vi "TDC_DAQV32_Paralled_muon.vi"(7 "address":string[](array[string])=["192.168.10.20"], 8 "error in (no error)":errorcluster, 9 "stop":bool=TRUE, 10 "save data":bool=TRUE, 11 "SMA mode":bool=TRUE) -> (0 "error out 3":errorcluster, 2 "csv path":path=path "G:/tdc/2017/data/test_20250326_071915.csv", 3 "rate":dbl=0.8977001365215763)   [LabVIEW 2017]
uses:
  gloabal.vi
  <vilib>/Utility/file.llb/Write Delimited Spreadsheet (DBL).vi
  <vilib>/Utility/file.llb/Write Delimited Spreadsheet (I64).vi
panel:
  in  "append csv 2":bool=TRUE
  out "accumulation":u32[][](array[numeric])
  out "pmt trigger rate":u32[](array[numeric])=[42662, 42662, 42662, 42662, 42662, 42662, 42662, 42662, 42662, 42662, 42662, 42662, 42662, 42662, 42662, 42662, 42662, 42662, 42662, 42662, 42662, 42662, 42662, 42662, 42662, 42662, 42662, 42662, 42662, 42662, 42662, 42662, 42662, 42662, 42662, 42662, 42662, 42662, 42662, 42662, 42662, 42662, 42662, 42662, 42662, 42662, 42662, 42662, 42662, 42662, 42662, 42662, 42662, 42662, 42662, 42662, 42662, 42662, 42662, 42662, 42662, 42662, 42662, 42662]
  out "event":u32[](array[numeric])=[26391, 26391, 26391, 26391, 26391, 26391, 26391, 26391, 26391, 26391, 26391, 26391, 26391, 26391, 26391, 26391, 26391, 26391, 26391, 26391, 26391, 26391, 26391, 26391, 26390, 26390, 26390, 26390, 26390, 26390, 26390, 26390, 26390, 26390, 26390, 26390, 26390, 26390, 26390, 26390, 26390, 26390, 26390, 26390, 26390, 26390, 26390, 26390, 26390, 26390, 26390, 26390, 26390, 26390, 26390, 26390, 26390, 26390, 26390, 26390, 26390, 26390, 26390, 26390, 26390, 26390, 26390, 26390, 26390, 26390, 26390, 26390, 26390, 26390, 26390, 26390, 26390, 26390, 26390, 26390, 26390, 26390, 26390, 26390, 26390, 26390, 26390, 26390, 26390, 26390, 26390, 26390, 26390, 26390, 26390, 26390, 26390, 26390, 26390, 26390, 26390, 26390, 26390, 26390, 26390, 26390, 26390, 26390, 26390, 26390, 26390, 26390, 26390, 26390, 26390, 26390, 26390, 26390, 26390, 26390, 26390, 26390, 26390, 26390, 26390, 26390, 26390, 26390]
  in  "calib_file":path=path "G:/tdc/2017/data/test_20250313_032748_codeDensity.csv" caption="文件路径 （空时为对话框）"
  in  "use_calib_file":bool
  out "cal 3":u32[](graph)=[0, 0, 0, 0, 0, 0, 0, 0, 0, 0, 0, 0, 0, 0, 0, 0, 0, 0, 0, 0, 0, 0, 0, 0, 0, 0, 0, 0, 0, 0, 0, 0, 0, 0, 0, 0, 0, 0, 0, 0, 0, 0, 0, 0, 0, 0, 0, 0, 0, 0, 0, 0, 0, 0, 0, 0, 0, 0, 0, 0, 0, 0, 0, 0, 0, 0, 0, 0, 0, 0, 0, 0, 0, 0, 0, 0, 0, 0, 0, 0, 0, 0, 0, 0, 0, 0, 0, 0, 0, 0, 0, 0, 0, 0, 0, 0, 0, 0, 0, 0, 0, 0, 0, 0, 0, 0, 0, 0, 0, 0, 0, 0, 0, 0, 0, 0, 0, 0, 0, 0, 0, 0, 0, 0, 0, 0, 0, 0, 0, 0, 0, 0, 0, 0, 0, 0, 0, 0, 0, 0, 0, 0, 0, 0, 0, 0, 0, 0, 0, 0, 0, 0, 0, 0, 0, 0, 0, 0, 0, 0, 0, 0, 0, 0, 0, 15, 3, 1, 14, 3, 31, 20, 16, 6, 1, 18, 12, 4, 29, 10, 8, 29, 2, 14, 4, 25, 7, 24, 4, 0, 1, 5, 8, 18, 22, 0, 4, 5, 0, 12, 9, 9, 20, 21, 4, 10, 13, 5, 21, 13, 14, 2, 6, 13, 1, 3, 5, 10, 20, 2, 3, 4, 3, 4, 2, 20, 13, 2, 5, 1, 3, 12, 4, 1, 14, 7, 5, 4, 1, 10, 2, 21, 14, 2, 5, 10, 4, 0, 11, 19, 6, 4, 1, 37, 1, 4, 2, 1, 10, 13, 4, 8, 10, 6, 9, 2, 0, 6, 8, 12, 3, 21, 5, 7, 8, 2, 3, 7, 17, 6, 5, 6, 4, 6, 0, 2, 1, 3, 10, 33, 7, 2, 6, 3, 7, 3, 2, 0, 12, 10, 11, 13, 13, 7, 3, 9, 6, 16, 0, 13, 5, 6, 3, 0, 5, 5, 7, 1, 10, 7, 13, 14, 5, 1, 12, 7, 1, 10, 2, 1, 14, 18, 13, 11, 4, 6, 9, 22, 11, 9, 2, 2, 8, 14, 4, 4, 6, 12, 13, 3, 9, 5, 5, 1, 5, 11, 18, 3, 0, 5, 4, 6, 7, 6, 1, 13, 5, 1, 2, 2, 1, 4, 12, 7, 3, 2, 3, 9, 11, 1, 20, 3, 4, 5, 5, 3, 5, 8, 5, 3, 26, 14, 6, 1, 3, 12, 12, 4, 23, 10, 3, 4, 4, 10, 3, 5, 4, 2, 14, 5, 15, 20, 1, 5, 1, 20, 6, 1, 3, 13, 21, 12, 7, 4, 1, 5, 30, 11, 2, 4, 0, 12, 7, 10, 3, 2, 25, 6, 1, 3, 6, 3, 8, 37, 4, 6, 2, 2, 4, 3, 5, 6, 13, 6, 9, 22, 1, 3, 7, 7, 4, 8, 33, 2, 1, 15, 3, 8, 23, 21, 2, 2, 27, 13, 3, 5, 10, 4, 18, 5, 5, 8, 0, 1, 8, 12, 4, 3, 0, 4, 8, 4, 7, 4, 2, 11, 13, 3, 0, 7, 5, 3, 4, 8, 4, 20, 2, 13, 4, 8, 6, 17, 4, 2, 1, 15, 2, 15, 5, 19, 0, 4, 15, 4, 16, 11, 1, 16, 4, 6, 6, 5, 7, 3, 9, 15, 3, 6, 3, 13, 5, 7, 3, 27, 2, 0, 21, 1, 4, 1, 4, 5, 3, 10, 7, 3, 6, 4, 18, 21, 7, 6, 7, 7, 12, 6, 9, 8, 11, 12, 13, 2, 2, 5, 4, 7, 52, 3, 5, 8, 7, 10, 4, 4, 6, 5, 18, 0, 3, 6, 1, 9, 5, 19, 13, 24, 12, 4, 4, 15, 6, 41, 3, 8, 5, 17, 26, 8, 7, 20, 2, 5, 12, 10, 10, 12, 9, 17, 6, 3, 1, 5, 3, 7, 8, 4, 10, 5, 10, 7, 1, 2, 14, 7, 25, 3, 0, 0, 0, 5, 21, 8, 14, 4, 10, 2, 3, 2, 4, 8, 12, 3, 6, 8, 3, 4, 3, 20, 5, 6, 7, 8, 11, 2, 8, 6, 5, 15, 17, 10, 10, 3, 3, 9, 18, 7, 7, 3, 5, 5, 5, 2, 2, 2, 4, 1, 0, 42, 3, 14, 4, 3, 5, 2, 7, 4, 2, 7, 5, 22, 4, 3, 17, 3, 5, 8, 19, 7, 5, 0, 3, 4, 10, 1, 8, 2, 2, 13, 23, 4, 9, 5, 0, 0, 0, 27, 2, 16, 11, 15, 3, 0, 18, 2, 8, 29, 19, 6, 7, 2, 6, 12, 1, 13, 2, 7, 5, 11, 8, 5, 6, 6, 19, 2, 4, 0, 7, 22, 13, 3, 7, 3, 8, 11, 0, 3, 26, 6, 5, 5, 6, 4, 10, 17, 16, 4, 3, 4, 3, 4, 21, 8, 10, 10, 7, 0, 9, 9, 2, 10, 10, 2, 9, 9, 4, 14, 5, 5, 4, 18, 6, 3, 0, 4, 1, 20, 2, 33, 4, 1, 2, 1, 20, 6, 3, 11, 10, 2, 1, 13, 9, 6, 1, 0, 0, 0, 0, 0, 0, 0, 0, 0, 0, 0, 0, 0, 0, 0, 0, 0, 0, 0, 0, 0, 0, 0, 0, 0, 0, 0, 0, 0, 0, 0, 0, 0, 0, 0, 0, 0, 0, 0, 0, 0, 0, 0, 0, 0, 0, 0, 0, 0, 0, 0, 0, 0, 0, 0, 0, 0, 0, 0, 0, 0, 0, 0, 0, 0, 0, 0, 0, 0, 0, 0, 0, 0, 0, 0, 0, 0, 0, 0, 0, 0, 0, 0, 0, 0, 0, 0, 0, 0, 0, 0, 0, 0, 0, 0, 0, 0, 0, 0, 0, 0, 0, 0, 0, 0, 0, 0, 0, 0, 0, 0, 0, 0, 0, 0, 0, 0, 0, 0, 0, 0, 0, 0, 0, 0, 0, 0, 0, 0, 0, 0, 0, 0, 0, 0, 0, 0, 0, 0, 0, 0, 0, 0, 0, 0, 0, 0, 0, 0, 0, 0, 0, 0, 0, 0, 0, 0, 0, 0, 0, 0, 0, 0, 0, 0, 0, 0, 0, 0, 0, 0, 0, 0, 0, 0, 0, 0, 0, 0, 0, 0, 0, 0, 0, 0, 0, 0, 0, 0, 0, 0, 0, 0, 0, 0, 0, 0, 0, 0, 0, 0, 0, 0, 0, 0, 0, 0, 0, 0, 0, 0, 0, 0, 0, 0, 0, 0, 0, 0, 0, 0, 0, 0, 0, 0, 0, 0, 0, 0, 0, 0, 0, 0, 0, 0, 0, 0, 0, 0, 0, 0, 0, 0, 0, 0, 0, 0, 0, 0, 0, 0, 0, 0, 0, 0, 0, 0, 0, 0, 0, 0, 0, 0, 0, 0, 0, 0, 0, 0, 0, 0, 0, 0, 0, 0, 0, 0, 0, 0, 0, 0, 0, 0, 0, 0, 0, 0, 0, 0, 0, 0, 0, 0, 0, 0, 0, 0, 0, 0, 0, 0, 0, 0, 0, 0, 0, 0, 0, 0, 0, 0, 0, 0, 0, 0, 0, 0, 0, 0, 0, 0, 0, 0, 0, 0, 0, 0, 0, 0, 0, 0, 0, 0, 0, 0, 0, 0, 0, 0, 0, 0, 0, 0, 0, 0, 0, 0, 0, 0, 0, 0, 0, 0, 0, 0, 0, 0, 0, 0, 0, 0, 0, 0, 0, 0, 0, 0, 0, 0, 0, 0, 0, 0, 0, 0, 0, 0, 0, 0, 0, 0, 0, 0, 0, 0, 0, 0, 0, 0, 0, 0, 0, 0, 0, 0, 0, 0, 0, 0, 0, 0, 0, 0, 0, 0, 0, 0, 0, 0, 0, 0, 0, 0, 0, 0, 0, 0, 0, 0, 0, 0, 0, 0, 0, 0, 0, 0, 0, 0, 0, 0, 0, 0, 0, 0, 0, 0, 0, 0, 0, 0, 0, 0, 0, 0, 0, 0, 0, 0, 0, 0, 0, 0, 0, 0, 0, 0, 0, 0, 0, 0, 0, 0, 0, 0, 0, 0, 0, 0, 0, 0, 0, 0, 0, 0, 0, 0, 0, 0, 0, 0, 0, 0, 0, 0, 0, 0, 0, 0, 0, 0, 0, 0, 0, 0, 0, 0, 0, 0, 0, 0, 0, 0, 0, 0, 0, 0, 0, 0, 0, 0, 0, 0, 0, 0, 0, 0, 0, 0, 0, 0, 0, 0, 0, 0, 0, 0, 0, 0, 0, 0, 0, 0, 0, 0, 0, 0, 0, 0, 0, 0, 0, 0, 0, 0, 0, 0, 0, 0, 0, 0, 0, 0, 0, 0, 0, 0, 0, 0, 0, 0, 0, 0, 0, 0, 0, 0, 0, 0, 0, 0, 0, 0, 0, 0, 0, 0, 0, 0, 0, 0, 0, 0, 0, 0, 0, 0, 0, 0, 0, 0, 0, 0, 0, 0, 0, 0, 0, 0, 0, 0, 0, 0, 0, 0, 0, 0, 0, 0, 0, 0, 0, 0, 0, 0, 0, 0, 0, 0, 0, 0, 0, 0, 0, 0, 0, 0, 0, 0, 0, 0, 0, 0, 0, 0, 0, 0, 0, 0, 0, 0, 0, 0, 0, 0, 0, 0, 0, 0, 0, 0, 0, 0, 0, 0, 0, 0, 0, 0, 0, 0, 0, 0, 0, 0, 0, 0, 0, 0, 0, 0, 0, 0, 0, 0, 0, 0, 0, 0, 0, 0, 0, 0, 0, 0, 0, 0, 0, 0, 0, 0, 0, 0, 0, 0, 0, 0, 0, 0, 0, 0, 0, 0, 0, 0, 0, 0, 0, 0, 0, 0, 0, 0, 0, 0, 0, 0, 0, 0, 0, 0, 0, 0, 0, 0, 0, 0, 0, 0, 0, 0, 0, 0, 0, 0, 0, 0, 0, 0, 0, 0, 0, 0, 0, 0, 0, 0, 0, 0, 0, 0, 0, 0, 0, 0, 0, 0, 0, 0, 0, 0, 0, 0, 0, 0, 0, 0, 0, 0, 0, 0, 0, 0, 0, 0, 0, 0, 0, 0, 0, 0, 0, 0, 0, 0, 0, 0, 0, 0, 0, 0, 0, 0, 0, 0, 0, 0, 0, 0, 0, 0, 0, 0, 0, 0, 0, 0, 0, 0, 0, 0, 0, 0, 0, 0, 0, 0, 0, 0, 0, 0, 0, 0, 0, 0, 0, 0, 0, 0, 0, 0, 0, 0, 0, 0, 0, 0, 0, 0, 0, 0, 0, 0, 0, 0, 0, 0, 0, 0, 0, 0, 0, 0, 0, 0, 0, 0, 0, 0, 0, 0, 0, 0, 0, 0, 0, 0, 0, 0, 0, 0, 0, 0, 0, 0, 0, 0, 0, 0, 0, 0, 0, 0, 0, 0, 0, 0, 0, 0, 0, 0, 0, 0, 0, 0, 0, 0, 0, 0, 0, 0, 0, 0, 0, 0, 0, 0, 0, 0, 0, 0, 0, 0, 0, 0, 0, 0, 0, 0, 0, 0, 0, 0, 0, 0, 0, 0, 0, 0, 0, 0, 0, 0, 0, 0, 0, 0, 0, 0, 0, 0, 0, 0, 0, 0, 0, 0, 0, 0, 0, 0, 0, 0, 0, 0, 0, 0, 0, 0, 0, 0, 0, 0, 0, 0, 0, 0, 0, 0, 0, 0, 0, 0, 0, 0, 0, 0, 0, 0, 0, 0, 0, 0, 0, 0, 0, 0, 0, 0, 0, 0, 0, 0, 0, 0, 0, 0, 0, 0, 0, 0, 0, 0, 0, 0, 0, 0, 0, 0, 0, 0, 0, 0, 0, 0, 0, 0, 0, 0, 0, 0, 0, 0, 0, 0, 0, 0, 0, 0, 0, 0, 0, 0, 0, 0, 0, 0, 0, 0, 0, 0, 0, 0, 0, 0, 0, 0, 0, 0, 0, 0, 0, 0, 0, 0, 0, 0, 0, 0, 0, 0, 0, 0, 0, 0, 0, 0, 0, 0, 0, 0, 0, 0, 0, 0, 0, 0, 0, 0, 0, 0, 0, 0, 0, 0, 0, 0, 0, 0, 0, 0, 0, 0, 0, 0, 0, 0, 0, 0, 0, 0, 0, 0, 0, 0, 0, 0, 0, 0, 0, 0, 0, 0, 0, 0, 0, 0, 0, 0, 0, 0, 0, 0, 0, 0, 0, 0, 0, 0, 0, 0, 0, 0, 0, 0, 0, 0, 0, 0, 0, 0, 0, 0, 0, 0, 0, 0, 0, 0, 0, 0, 0, 0, 0, 0, 0, 0, 0, 0, 0, 0, 0, 0, 0, 0, 0, 0, 0, 0, 0, 0, 0, 0, 0, 0, 0, 0, 0, 0, 0, 0, 0, 0, 0, 0, 0, 0, 0, 0, 0, 0, 0, 0, 0, 0, 0, 0, 0, 0, 0, 0, 0, 0, 0, 0, 0, 0, 0, 0, 0, 0, 0, 0, 0, 0, 0, 0, 0, 0, 0, 0, 0, 0, 0, 0]
  out "second stamp":u64
  in  "coarse counter width":u16(ring) items=["29", "48"]
  out "name (unnamed)":string
  out "error out 5":errorcluster
  in  "timeout":dbl=30000.0
  out "DAC":dbl=8094.0
  out "Out":u8=3 format="%.0x"
  out "coarse":u64=454674664 format="%x"
  in  "gps":bool
  out "Year":string="2025"
  in  "factor":i32=128
  in  "displayCR":bool=TRUE
  in  "Counter Setting":dbl=100000.0 format="%#_13g"
  in  "replace dat":bool
  in  "append csv":bool=TRUE
  out "element":string
  out "fine":u64=621 format="%x"
  in  "UDP Config":bool=TRUE
  in  "data  path":path=path "G:/tdc/2017/data"
  out "cal 2":u64[](graph)
  in  "Thresholds (mV)":dbl[](array[numeric])=[580.0, 580.0, 580.0, 580.0, 600.0, 600.0, 600.0, 600.0, 580.0, 580.0, 600.0, 600.0, 600.0, 600.0, 600.0, 600.0, 580.0, 580.0, 600.0, 600.0, 600.0, 600.0, 600.0, 600.0, 580.0, 580.0, 600.0, 600.0, 600.0, 600.0, 600.0, 600.0, 600.0, 600.0, 600.0, 600.0, 600.0, 600.0, 600.0, 600.0, 600.0, 600.0, 600.0, 600.0, 600.0, 600.0, 600.0, 600.0, 600.0, 600.0, 600.0, 600.0, 600.0, 600.0, 600.0, 600.0, 600.0, 600.0, 600.0, 600.0, 600.0, 600.0, 600.0, 600.0]
  out "error out 2":errorcluster
  in  "display":bool=TRUE
  in  "Thresholds":dbl=-0.03
  in  "one key for threshold":bool=TRUE
  in  "RST":bool
  in  "通道数量":i32=128
  out "Cal Table":u32[](array[numeric])=[100002, 100002, 100002, 100002, 100002, 100002, 100002, 100002, 100002, 100002, 100002, 100002, 100002, 100002, 100002, 100002, 100002, 100002, 100002, 100002, 100002, 100002, 100002, 100002, 100002, 100002, 100002, 100002, 100002, 100002, 100002, 100002, 100002, 100002, 100002, 100002, 100002, 100002, 100002, 100002, 100002, 100002, 100002, 100002, 100002, 100002, 100002, 100002, 100002, 100002, 100002, 100002, 100002, 100002, 100002, 100002, 100002, 100002, 100002, 100002, 100002, 100002, 100002, 100002, 100002, 100002, 100002, 100002, 100002, 100002, 100002, 100002, 100002, 100002, 100002, 100002, 100002, 100002, 100002, 100002, 100002, 100002, 100002, 100002, 100002, 100002, 100002, 100002, 100002, 100002, 100002, 100002, 100002, 100002, 100002, 100002, 100002, 100002, 100002, 100002, 100002, 100002, 100002, 100002, 100002, 100002, 100002, 100002, 100002, 100002, 100002, 100002, 100002, 100002, 100002, 100002, 100002, 100002, 100002, 100002, 100002, 100002, 100002, 100002, 100002, 100002, 100002, 100002]
  in  "channel for cal":i32
  out "channel number":u64
  out "Calibration Counter":i32=100000
  out "Event index":i32=97959
  out "cal":i64[](graph)=[0, 0, 0, 0, 0, 0, 0, 0, 0, 0, 0, 0, 0, 0, 0, 0, 0, 0, 0, 0, 0, 0, 0, 0, 0, 0, 0, 0, 0, 0, 0, 0, 0, 0, 0, 0, 0, 0, 0, 0, 0, 0, 0, 0, 0, 0, 0, 0, 0, 0, 0, 0, 0, 0, 0, 0, 0, 0, 0, 0, 0, 0, 0, 0, 0, 0, 0, 0, 0, 0, 0, 0, 0, 0, 0, 0, 0, 0, 0, 0, 0, 0, 0, 0, 0, 0, 0, 0, 0, 0, 0, 0, 0, 0, 0, 0, 0, 0, 0, 0, 0, 0, 0, 0, 0, 0, 0, 0, 0, 0, 0, 0, 0, 0, 0, 0, 0, 0, 0, 0, 0, 0, 0, 0, 0, 0, 0, 0, 0, 0, 0, 0, 0, 0, 0, 0, 0, 0, 0, 470, 444, 62, 95, 368, 213, 276, 85, 576, 217, 42, 61, 213, 135, 123, 54, 784, 126, 136, 66, 62, 275, 126, 450, 146, 386, 84, 83, 84, 62, 253, 57, 502, 202, 53, 85, 337, 200, 58, 83, 413, 78, 317, 61, 148, 133, 102, 48, 479, 56, 216, 194, 40, 112, 63, 351, 135, 190, 64, 93, 227, 93, 232, 114, 257, 110, 101, 159, 65, 42, 76, 54, 50, 44, 34, 359, 299, 101, 217, 71, 56, 60, 35, 455, 55, 67, 165, 158, 73, 196, 324, 124, 309, 54, 58, 141, 218, 413, 311, 78, 256, 130, 114, 294, 134, 50, 55, 28, 324, 26, 45, 329, 65, 45, 61, 116, 74, 323, 82, 79, 76, 85, 71, 72, 82, 187, 243, 204, 247, 62, 155, 92, 292, 69, 301, 30, 91, 225, 164, 64, 174, 87, 39, 48, 55, 627, 68, 232, 183, 142, 127, 63, 54, 315, 53, 77, 55, 116, 317, 193, 216, 219, 230, 235, 57, 55, 234, 42, 47, 57, 143, 358, 59, 153, 234, 79, 52, 154, 36, 378, 66, 258, 119, 74, 244, 119, 148, 52, 254, 251, 157, 243, 71, 102, 77, 477, 87, 292, 296, 458, 55, 177, 38, 31, 35, 56, 381, 340, 362, 127, 55, 39, 79, 277, 44, 40, 62, 68, 250, 24, 117, 88, 162, 67, 344, 104, 160, 92, 123, 54, 92, 68, 278, 168, 79, 408, 53, 38, 58, 56, 61, 51, 226, 81, 206, 224, 500, 85, 60, 69, 185, 271, 118, 166, 51, 65, 152, 192, 52, 91, 90, 286, 93, 314, 82, 82, 106, 261, 208, 80, 229, 101, 81, 224, 153, 256, 98, 36, 59, 67, 613, 43, 43, 40, 267, 68, 56, 271, 170, 98, 131, 79, 159, 86, 165, 217, 404, 83, 71, 135, 94, 174, 172, 48, 56, 441, 218, 102, 71, 139, 121, 137, 130, 148, 401, 140, 150, 182, 72, 207, 72, 62, 128, 217, 156, 471, 148, 53, 39, 329, 106, 142, 164, 131, 231, 54, 182, 112, 141, 281, 153, 313, 69, 72, 41, 181, 218, 56, 141, 81, 198, 63, 58, 241, 203, 104, 45, 40, 47, 205, 84, 42, 44, 387, 216, 158, 43, 59, 146, 97, 73, 100, 342, 95, 83, 88, 277, 184, 104, 53, 65, 275, 156, 245, 83, 62, 118, 206, 283, 48, 91, 102, 173, 63, 398, 66, 132, 65, 188, 274, 51, 53, 168, 132, 106, 221, 49, 50, 103, 174, 71, 211, 557, 53, 102, 53, 204, 86, 150, 145, 68, 211, 44, 81, 420, 104, 142, 288, 175, 62, 71, 473, 67, 134, 127, 170, 74, 65, 146, 161, 79, 106, 142, 273, 138, 369, 67, 79, 180, 264, 83, 430, 55, 98, 97, 181, 45, 247, 290, 174, 330, 59, 190, 39, 34, 33, 58, 203, 128, 109, 108, 82, 293, 87, 62, 98, 103, 58, 52, 46, 712, 43, 50, 133, 458, 172, 395, 40, 43, 159, 147, 158, 109, 667, 52, 38, 107, 336, 421, 194, 61, 296, 123, 176, 103, 87, 166, 71, 165, 673, 92, 58, 171, 158, 64, 62, 120, 117, 207, 128, 149, 55, 63, 80, 137, 395, 136, 100, 110, 227, 70, 132, 142, 66, 113, 419, 55, 35, 62, 201, 78, 444, 318, 150, 54, 241, 72, 45, 54, 112, 201, 339, 87, 74, 279, 84, 136, 156, 98, 295, 59, 372, 94, 109, 76, 101, 122, 109, 209, 266, 83, 153, 259, 425, 131, 78, 229, 112, 66, 144, 47, 42, 125, 91, 418, 268, 143, 61, 36, 57, 219, 95, 46, 200, 120, 424, 116, 180, 252, 147, 184, 183, 76, 123, 180, 296, 531, 86, 54, 63, 173, 311, 698, 101, 76, 70, 106, 88, 275, 465, 105, 160, 48, 44, 88, 334, 497, 123, 42, 60, 34, 296, 72, 68, 73, 141, 259, 79, 46, 57, 60, 92, 72, 9, 21, 0, 0, 0, 0, 0, 0, 0, 0, 0, 0, 0, 0, 0, 0, 0, 0, 0, 0, 0, 0, 0, 0, 0, 0, 0, 0, 0, 0, 0, 0, 0, 0, 0, 0, 0, 0, 0, 0, 0, 0, 0, 0, 0, 0, 0, 0, 0, 0, 0, 0, 0, 0, 0, 0, 0, 0, 0, 0, 0, 0, 0, 0, 0, 0, 0, 0, 0, 0, 0, 0, 0, 0, 0, 0, 0, 0, 0, 0, 0, 0, 0, 0, 0, 0, 0, 0, 0, 0, 0, 0, 0, 0, 0, 0, 0, 0, 0, 0, 0, 0, 0, 0, 0, 0, 0, 0, 0, 0, 0, 0, 0, 0, 0, 0, 0, 0, 0, 0, 0, 0, 0, 0, 0, 0, 0, 0, 0, 0, 0, 0, 0, 0, 0, 0, 0, 0, 0, 0, 0, 0, 0, 0, 0, 0, 0, 0, 0, 0, 0, 0, 0, 0, 0, 0, 0, 0, 0, 0, 0, 0, 0, 0, 0, 0, 0, 0, 0, 0, 0, 0, 0, 0, 0, 0, 0, 0, 0, 0, 0, 0, 0, 0, 0, 0, 0, 0, 0, 0, 0, 0, 0, 0, 0, 0, 0, 0, 0, 0, 0, 0, 0, 0, 0, 0, 0, 0, 0, 0, 0, 0, 0, 0, 0, 0, 0, 0, 0, 0, 0, 0, 0, 0, 0, 0, 0, 0, 0, 0, 0, 0, 0, 0, 0, 0, 0, 0, 0, 0, 0, 0, 0, 0, 0, 0, 0, 0, 0, 0, 0, 0, 0, 0, 0, 0, 0, 0, 0, 0, 0, 0, 0, 0, 0, 0, 0, 0, 0, 0, 0, 0, 0, 0, 0, 0, 0, 0, 0, 0, 0, 0, 0, 0, 0, 0, 0, 0, 0, 0, 0, 0, 0, 0, 0, 0, 0, 0, 0, 0, 0, 0, 0, 0, 0, 0, 0, 0, 0, 0, 0, 0, 0, 0, 0, 0, 0, 0, 0, 0, 0, 0, 0, 0, 0, 0, 0, 0, 0, 0, 0, 0, 0, 0, 0, 0, 0, 0, 0, 0, 0, 0, 0, 0, 0, 0, 0, 0, 0, 0, 0, 0, 0, 0, 0, 0, 0, 0, 0, 0, 0, 0, 0, 0, 0, 0, 0, 0, 0, 0, 0, 0, 0, 0, 0, 0, 0, 0, 0, 0, 0, 0, 0, 0, 0, 0, 0, 0, 0, 0, 0, 0, 0, 0, 0, 0, 0, 0, 0, 0, 0, 0, 0, 0, 0, 0, 0, 0, 0, 0, 0, 0, 0, 0, 0, 0, 0, 0, 0, 0, 0, 0, 0, 0, 0, 0, 0, 0, 0, 0, 0, 0, 0, 0, 0, 0, 0, 0, 0, 0, 0, 0, 0, 0, 0, 0, 0, 0, 0, 0, 0, 0, 0, 0, 0, 0, 0, 0, 0, 0, 0, 0, 0, 0, 0, 0, 0, 0, 0, 0, 0, 0, 0, 0, 0, 0, 0, 0, 0, 0, 0, 0, 0, 0, 0, 0, 0, 0, 0, 0, 0, 0, 0, 0, 0, 0, 0, 0, 0, 0, 0, 0, 0, 0, 0, 0, 0, 0, 0, 0, 0, 0, 0, 0, 0, 0, 0, 0, 0, 0, 0, 0, 0, 0, 0, 0, 0, 0, 0, 0, 0, 0, 0, 0, 0, 0, 0, 0, 0, 0, 0, 0, 0, 0, 0, 0, 0, 0, 0, 0, 0, 0, 0, 0, 0, 0, 0, 0, 0, 0, 0, 0, 0, 0, 0, 0, 0, 0, 0, 0, 0, 0, 0, 0, 0, 0, 0, 0, 0, 0, 0, 0, 0, 0, 0, 0, 0, 0, 0, 0, 0, 0, 0, 0, 0, 0, 0, 0, 0, 0, 0, 0, 0, 0, 0, 0, 0, 0, 0, 0, 0, 0, 0, 0, 0, 0, 0, 0, 0, 0, 0, 0, 0, 0, 0, 0, 0, 0, 0, 0, 0, 0, 0, 0, 0, 0, 0, 0, 0, 0, 0, 0, 0, 0, 0, 0, 0, 0, 0, 0, 0, 0, 0, 0, 0, 0, 0, 0, 0, 0, 0, 0, 0, 0, 0, 0, 0, 0, 0, 0, 0, 0, 0, 0, 0, 0, 0, 0, 0, 0, 0, 0, 0, 0, 0, 0, 0, 0, 0, 0, 0, 0, 0, 0, 0, 0, 0, 0, 0, 0, 0, 0, 0, 0, 0, 0, 0, 0, 0, 0, 0, 0, 0, 0, 0, 0, 0, 0, 0, 0, 0, 0, 0, 0, 0, 0, 0, 0, 0, 0, 0, 0, 0, 0, 0, 0, 0, 0, 0, 0, 0, 0, 0, 0, 0, 0, 0, 0, 0, 0, 0, 0, 0, 0, 0, 0, 0, 0, 0, 0, 0, 0, 0, 0, 0, 0, 0, 0, 0, 0, 0, 0, 0, 0, 0, 0, 0, 0, 0, 0, 0, 0, 0, 0, 0, 0, 0, 0, 0, 0, 0, 0, 0, 0, 0, 0, 0, 0, 0, 0, 0, 0, 0, 0, 0, 0, 0, 0, 0, 0, 0, 0, 0, 0, 0, 0, 0, 0, 0, 0, 0, 0, 0, 0, 0, 0, 0, 0, 0, 0, 0, 0, 0, 0, 0, 0, 0, 0, 0, 0, 0, 0, 0, 0, 0, 0, 0, 0, 0, 0, 0, 0, 0, 0, 0, 0, 0, 0, 0, 0, 0, 0, 0, 0, 0, 0, 0, 0, 0, 0, 0, 0, 0, 0, 0, 0, 0, 0, 0, 0, 0, 0, 0, 0, 0, 0, 0, 0, 0, 0, 0, 0, 0, 0, 0, 0, 0, 0, 0, 0, 0, 0, 0, 0, 0, 0, 0, 0, 0, 0, 0, 0, 0, 0, 0, 0, 0, 0, 0, 0, 0, 0, 0, 0, 0, 0, 0, 0, 0, 0, 0, 0, 0, 0, 0, 0, 0, 0, 0, 0, 0, 0, 0, 0, 0, 0, 0, 0, 0, 0, 0, 0, 0, 0, 0, 0, 0, 0, 0, 0, 0, 0, 0, 0, 0, 0, 0, 0, 0, 0, 0, 0, 0, 0, 0, 0, 0, 0, 0, 0, 0, 0, 0, 0, 0, 0, 0, 0, 0, 0, 0, 0, 0, 0, 0, 0, 0, 0, 0, 0, 0, 0, 0, 0, 0, 0, 0, 0, 0, 0, 0, 0, 0, 0, 0, 0, 0, 0, 0, 0, 0, 0, 0, 0, 0, 0, 0, 0, 0, 0, 0, 0, 0, 0, 0, 0, 0, 0, 0, 0, 0, 0, 0, 0, 0, 0, 0, 0, 0, 0, 0, 0, 0, 0, 0, 0, 0, 0, 0, 0, 0, 0, 0, 0, 0, 0, 0, 0, 0, 0, 0, 0, 0, 0, 0, 0, 0, 0, 0, 0, 0, 0, 0, 0, 0, 0, 0, 0, 0, 0, 0, 0, 0, 0, 0, 0, 0, 0, 0, 0, 0, 0, 0, 0, 0, 0, 0, 0, 0, 0, 0, 0, 0, 0, 0, 0, 0, 0, 0, 0, 0, 0, 0, 0, 0, 0, 0, 0, 0, 0, 0, 0, 0, 0, 0, 0, 0, 0, 0, 0, 0, 0, 0, 0, 0, 0, 0, 0, 0, 0, 0, 0, 0, 0, 0, 0, 0, 0, 0, 0, 0, 0, 0, 0, 0, 0, 0, 0, 0, 0, 0, 0, 0, 0, 0, 0, 0, 0, 0, 0, 0, 0, 0, 0, 0, 0, 0, 0, 0, 0, 0, 0, 0, 0, 0, 0, 0, 0, 0, 0, 0, 0, 0, 0, 0, 0, 0, 0, 0, 0, 0, 0, 0, 0, 0, 0, 0, 0, 0, 0, 0, 0, 0, 0, 0, 0, 0, 0, 0, 0, 0, 0, 0, 0, 0, 0, 0, 0, 0, 0, 0, 0, 0, 0, 0, 0, 0, 0, 0, 0, 0, 0, 0, 0, 0, 0, 0, 0, 0, 0, 0, 0, 0, 0, 0, 0]
  out "error out":errorcluster
  out "appended path":path=path "G:/tdc/2017/data/test_20250326_071915.dat"
  in  "filename":string="test"
  in  "Events":i32=110000 min=1
  in  "timeout (ms)":i32=10000
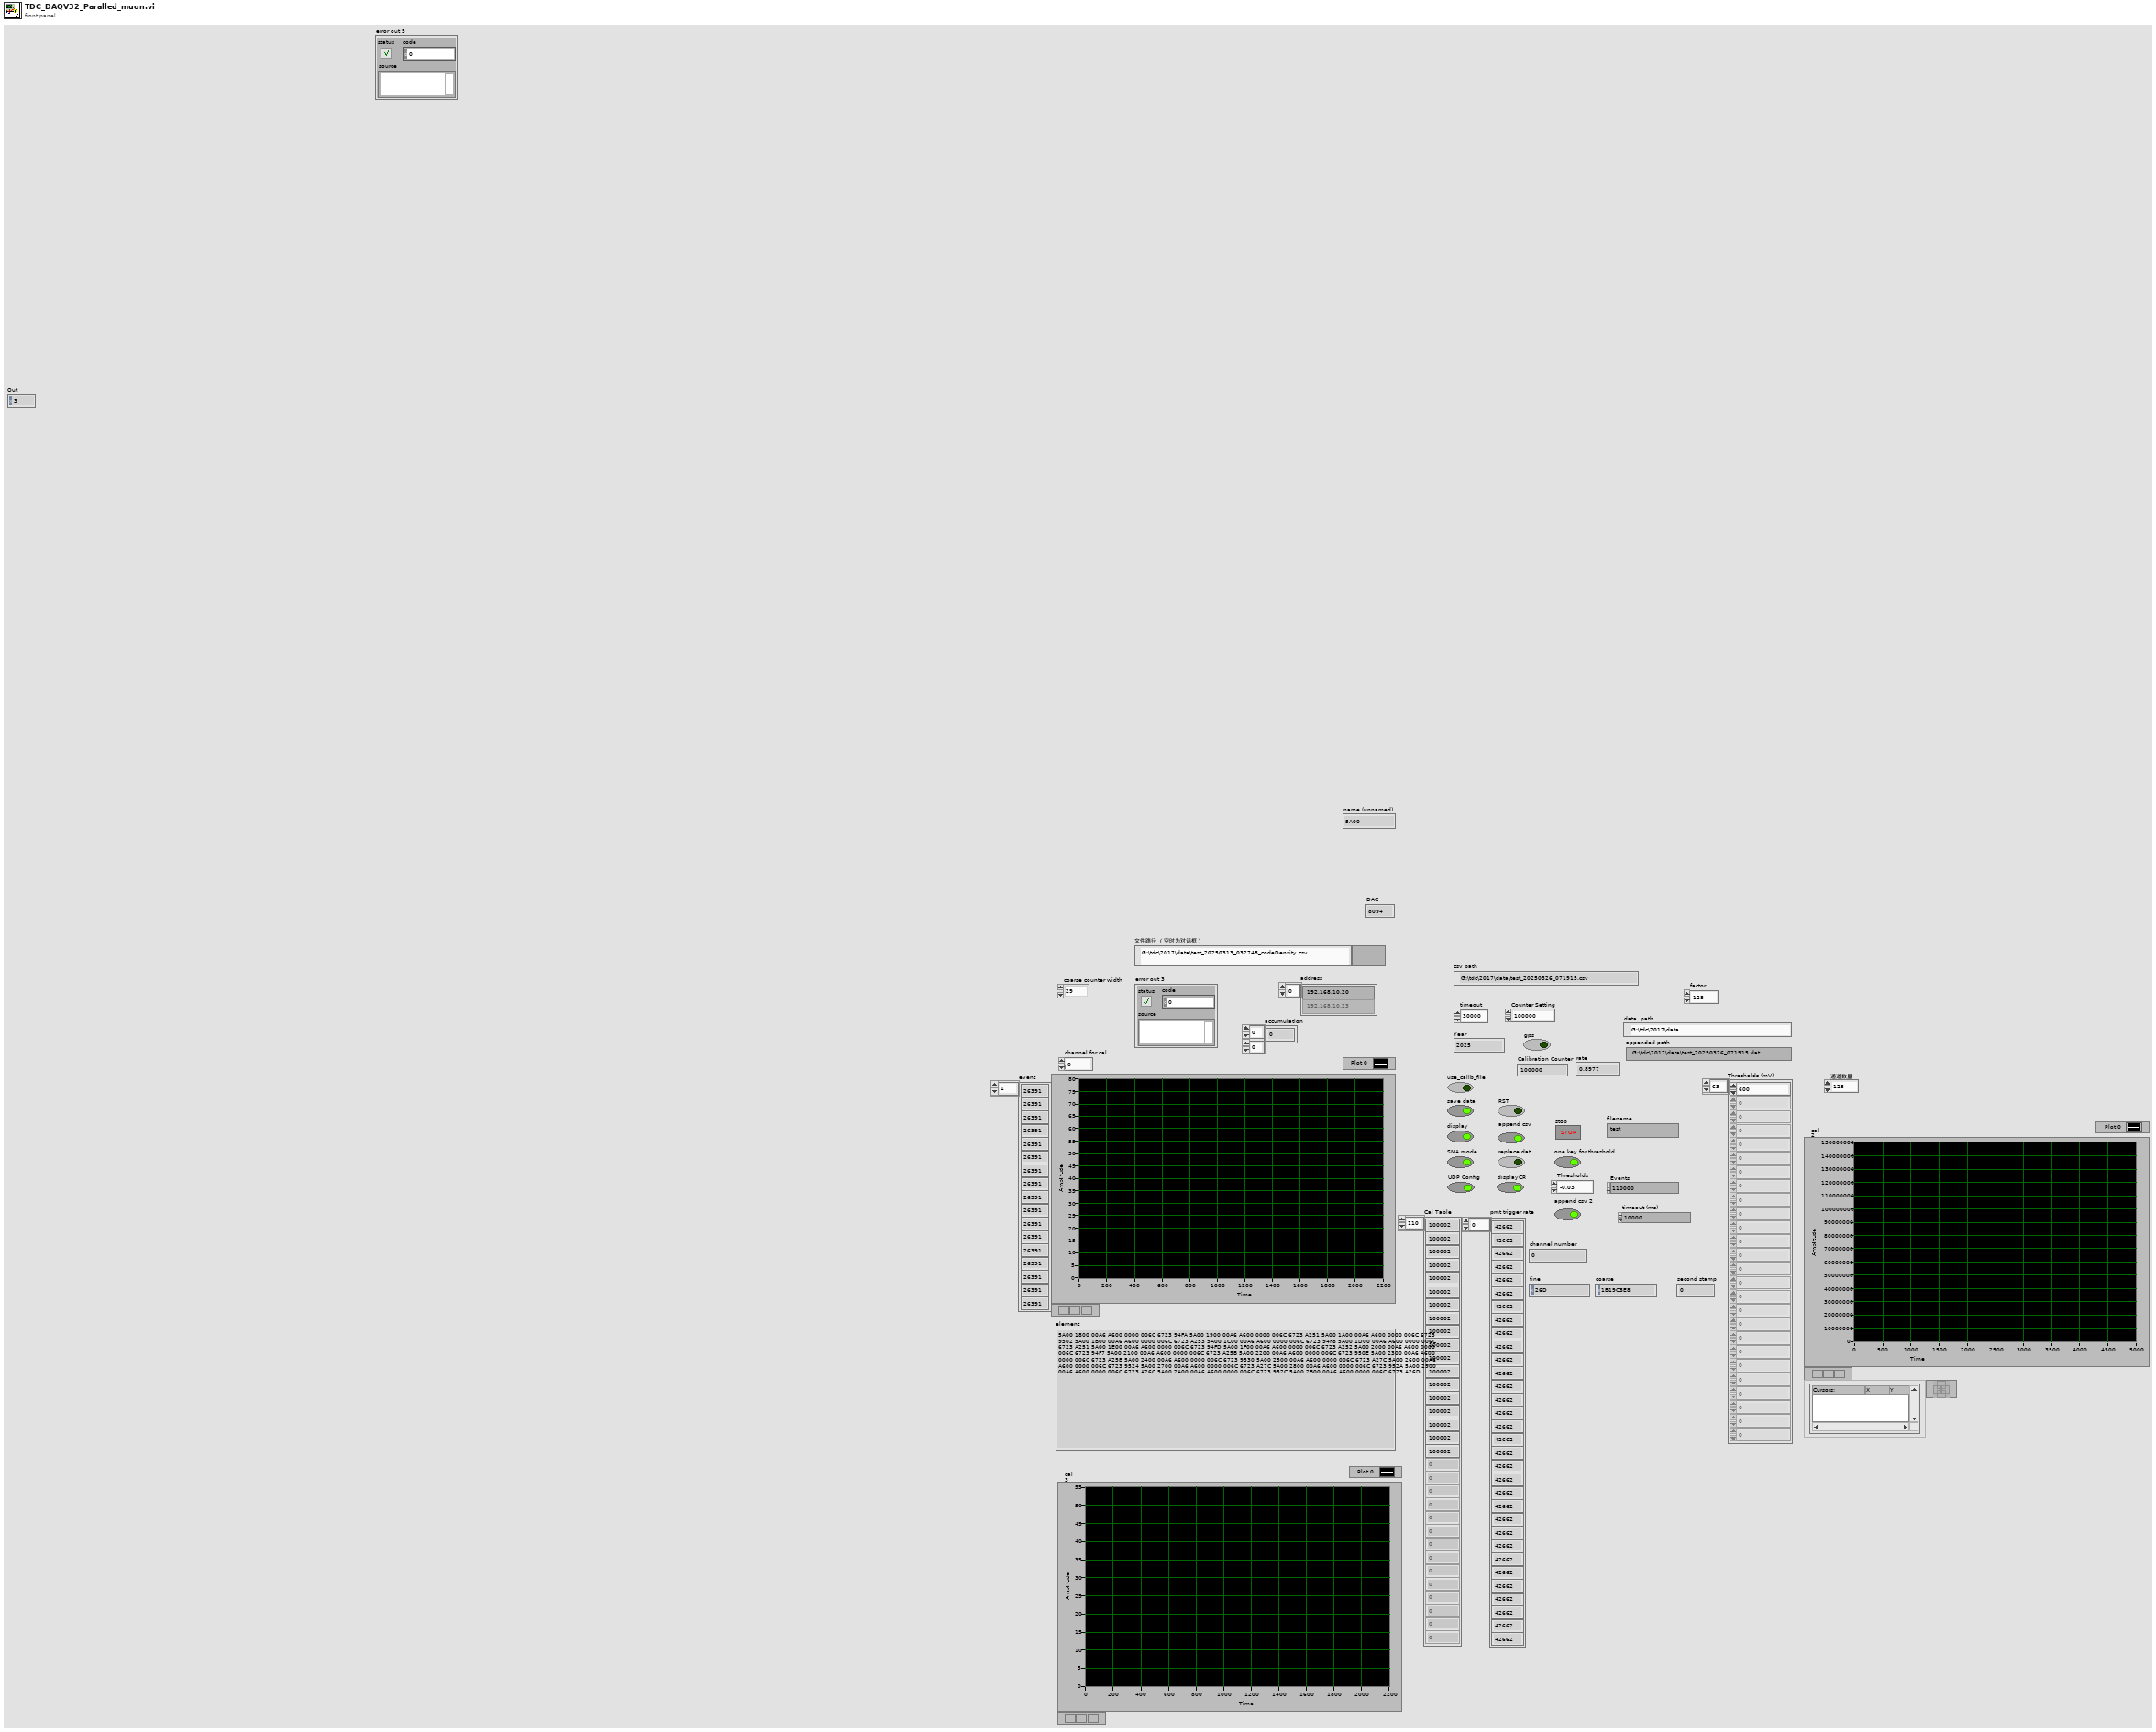
[diagram p1: front panel]
types:
  T1 = enum16{"open", "replace", "create", "open or create", "replace or create", "replace or create with confirmation"}
  T2 = enum16{"big-endian, network order", "native, host order", "little-endian"}
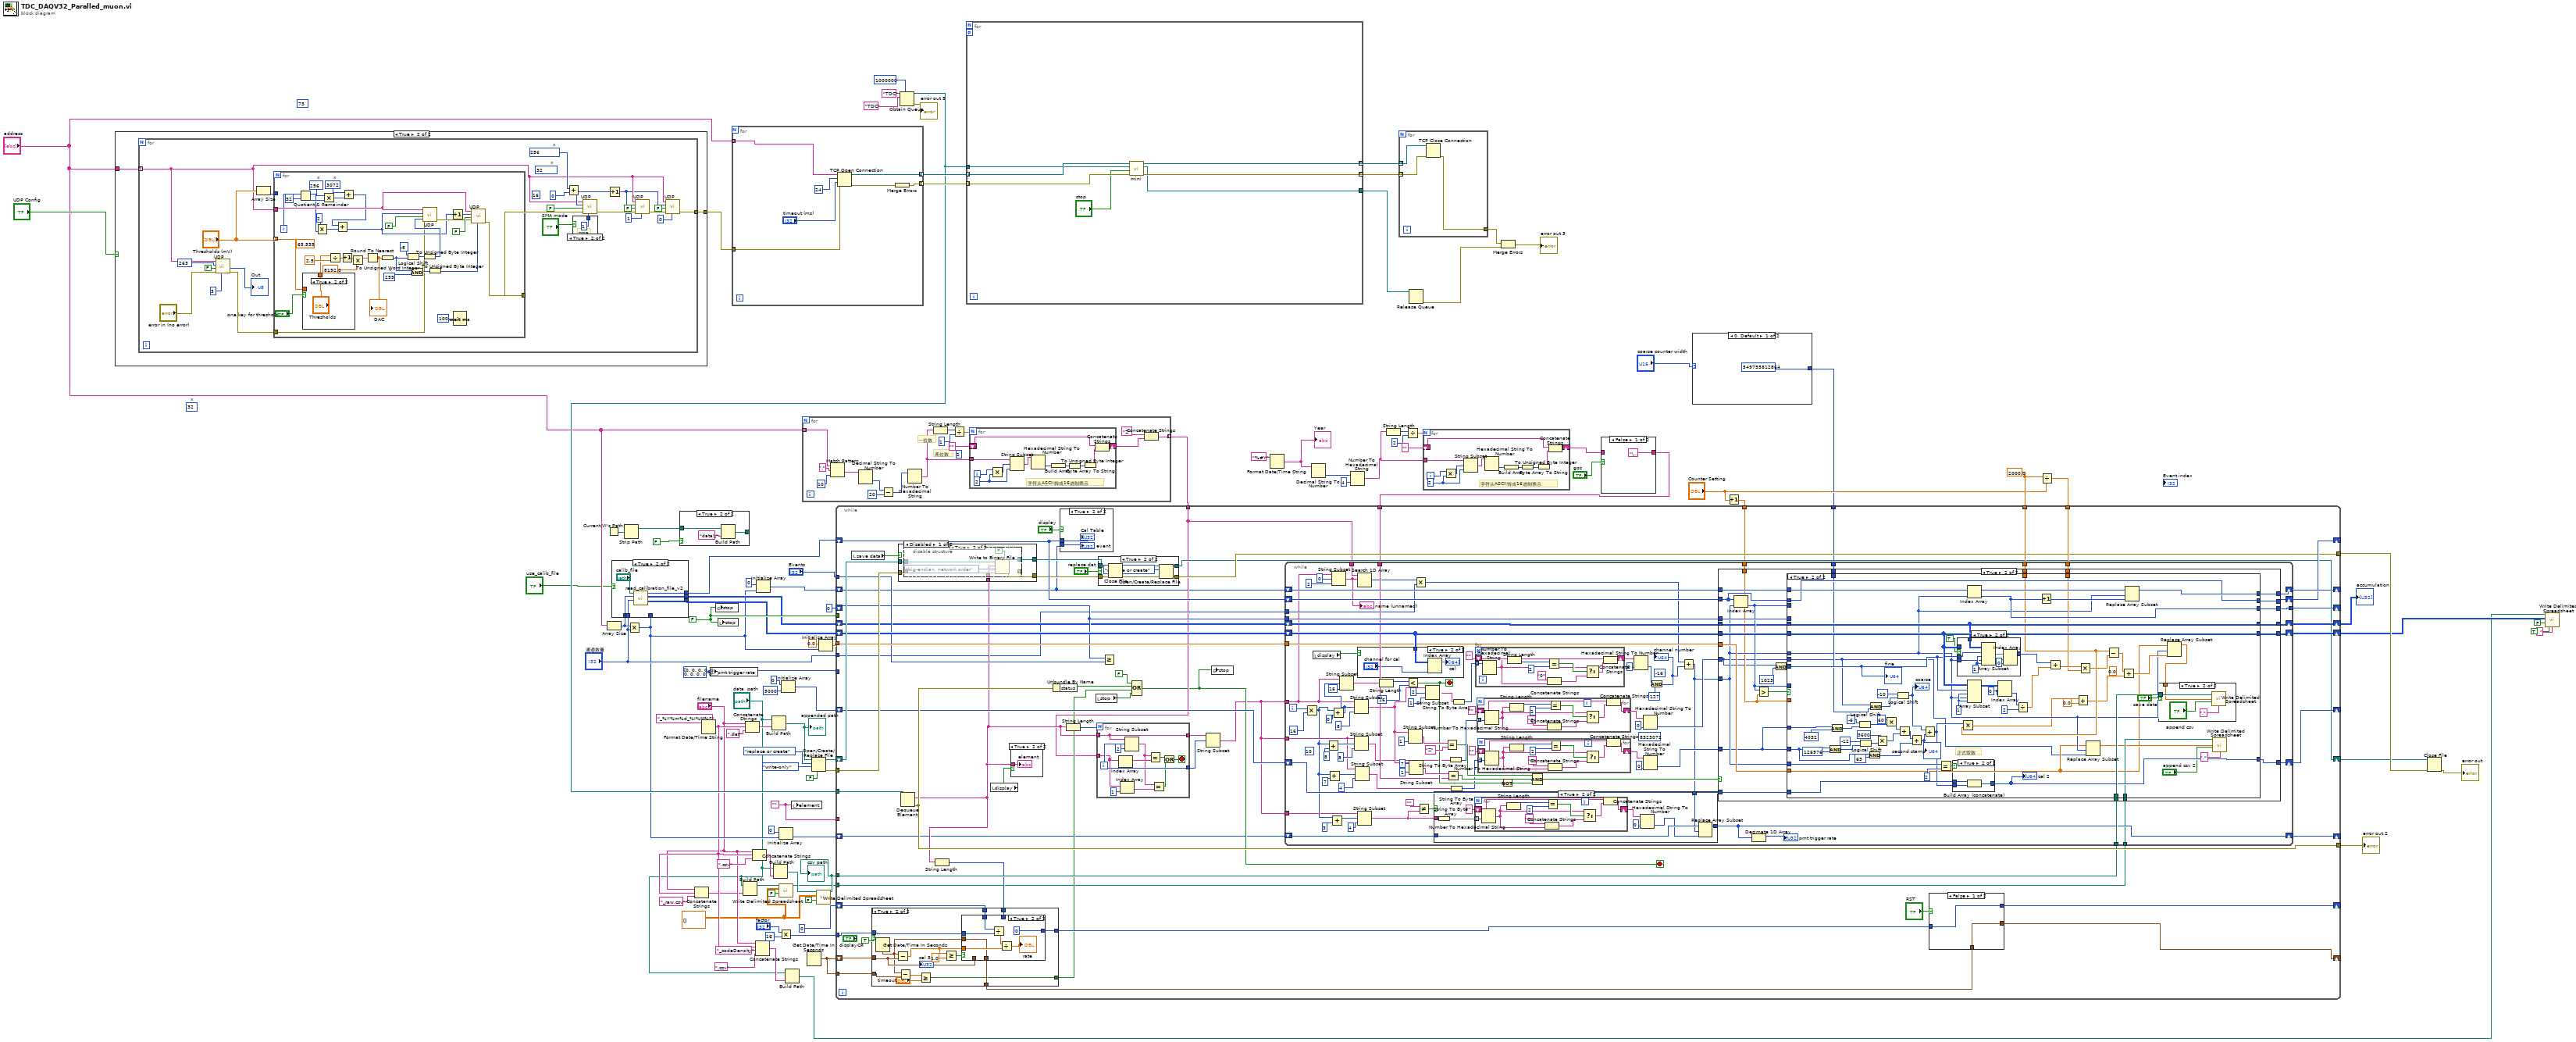
[diagram p0: block diagram]
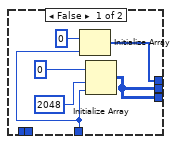
[diagram p2: hidden frame]
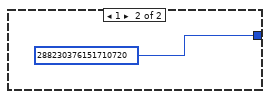
[diagram p3: hidden frame]
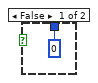
[diagram p6: hidden frame]
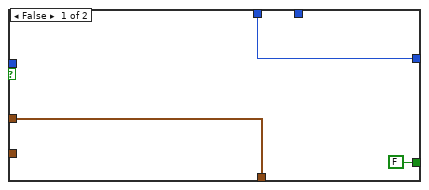
[diagram p13: hidden frame]
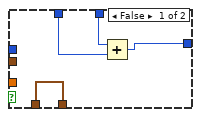
[diagram p14: hidden frame]
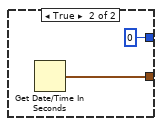
[diagram p16: hidden frame]
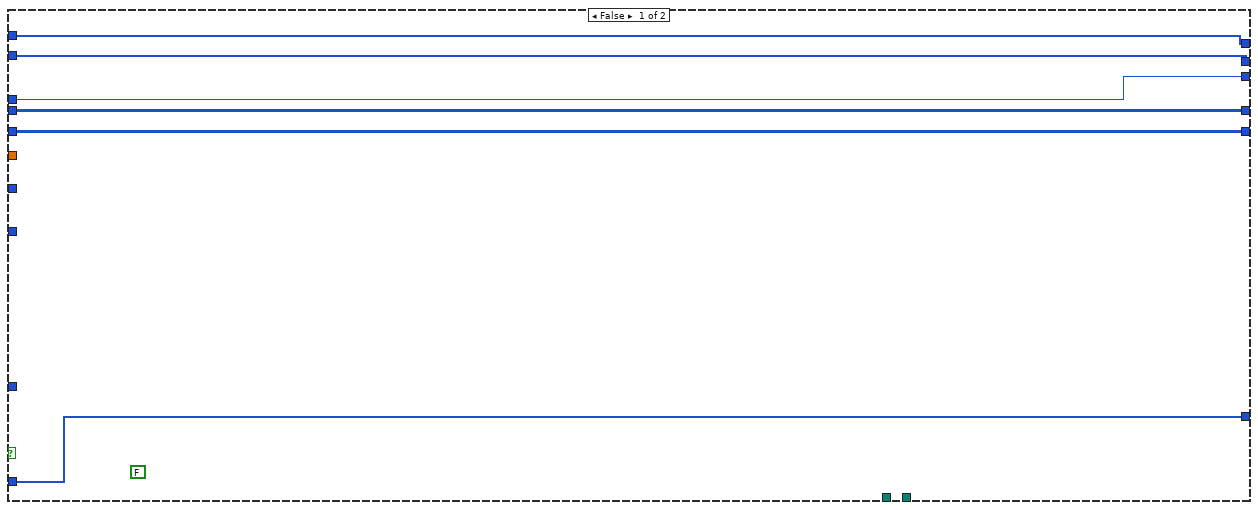
[diagram p19: hidden frame]
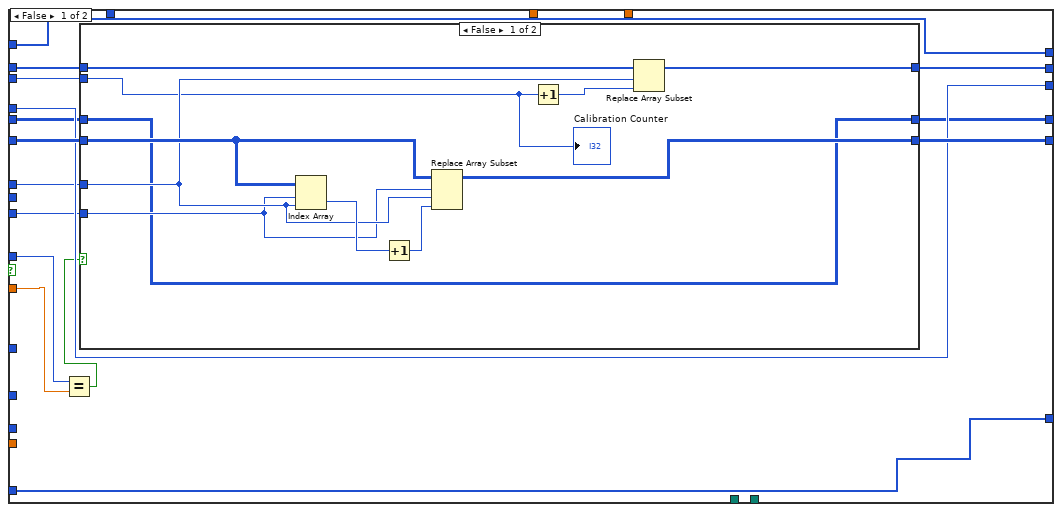
[diagram p20: hidden frame]
diagram:
  w11 = ""
  w12 = u32[] [0, 0, 0, 0, 0, 0, 0, 0, 0, 0, 0, 0, 0, 0, 0, 0, 0, 0, 0, 0, 0, 0, 0, 0, 0, 0, 0, 0, 0, 0, 0, 0, 0, 0, 0, 0, 0, 0, 0, 0, 0, 0, 0, 0, 0, 0, 0, 0, 0, 0, 0, 0, 0, 0, 0, 0, 0, 0, 0, 0, 0, 0, 0, 0] ("pmt trigger rate")
  (unwired) u32 73 ("Address")
  w63 = 2000.0 ("x")
  (unwired) u16 32  # x
  w25 = FALSE ("stop")
  w4 = dbl[][] [] ("2D data")
  n1 = case shown="True" "UDP Config" {
    tunnel: "address" -> [_ w101]
    tunnel: [_ w102] -> w30
    frame False {
    }
    frame True {
      n2 = for {
        tunnel: [w107] -> w102
        tunnel: w101 -> [w105] mode=indexing
        (unwired) u16 32  # x
        (unwired) u32 16 ("Address")
        w119 = u16 256  # x
        n3 = call "UDP.vi"("In"=u8 3, "error in (no error)"="error in (no error)", "Read (TRUE)"=FALSE, "Address"=u32 263, "IP address"=w105) -> ("error out"=w113:errorcluster, "Out"=→"Out":u8)  [unwired: 3 in, 1 out]
        n4 = Array Size(array="Thresholds (mV)") -> (size(s)=w122:i32)
        n5 = for {
          tunnel: w105 -> [w158]
          tunnel: "Thresholds (mV)" -> [w145] mode=indexing
          tunnel: [w148] -> w125
          tunnel: w122 -> [_]
          tunnel: w113 -> [w132]
          i -> [w140]
          (unwired) 65.535 ("y")
          w141 = u16 3072  # x
          w142 = u16 256  # x
          w154 = u16 255  # x
          n6 = Quotient & Remainder(x=w140, y=32) -> (x-y*floor(x/y)=w134:i32, floor(x/y)=w143:i32)
          n7 = case shown="True" "one key for threshold" {
            tunnel: [w164 "Thresholds"] -> w146
            tunnel: w145 -> [w164 _]
            frame False {
            }
            frame True {
            }
          }
          n8 = Multiply(x=2, y=w134) -> (x*y=w135:i32)
          n9 = Multiply(x=w142, y=w143) -> (x*y=w137:i32)
          n10 = Divide(x=w146, y=2.5) -> (x/y=w161:dbl)
          n11 = Increment(x=w161) -> (x+1=w131:dbl)
          n12 = Add(x=w141, y=w137) -> (x+y=w136:i32)
          n13 = Add(x=w136, y=w135) -> (x+y=w139:i32)
          n14 = Multiply(x=w131, y=8192.0) -> (x*y=w130:dbl)
          n15 = Round To Nearest(number=w130) -> (nearest integer value=w159:dbl)
          "DAC" <- w159
          n16 = To Unsigned Word Integer(number=w159) -> (unsigned 16bit integer=w150:u16)
          n17 = Logical Shift(y=i16 -8, x=w150) -> (x << y=w156:u16)
          n18 = And(x=w150, y=w154) -> (x .and. y?=w153:u16)
          n19 = To Unsigned Byte Integer(number=w156) -> (unsigned 8bit integer=w155:u8)
          n20 = call "UDP.vi"("In"=w155, "error in (no error)"=w132, "Read (TRUE)"=FALSE, "Address"=w139, "IP address"=w158) -> ("error out"=w149:errorcluster)  [unwired: 3 in, 2 out]
          n21 = To Unsigned Byte Integer(number=w153) -> (unsigned 8bit integer=w152:u8)
          n22 = Increment(x=w139) -> (x+1=w138:i32)
          n23 = Wait (ms)(milliseconds to wait=u32 100) -> ()  [unwired: 1 out]
          n24 = call "UDP.vi"("In"=w152, "error in (no error)"=w149, "Read (TRUE)"=FALSE, "Address"=w138, "IP address"=w158) -> ("error out"=w148:errorcluster)  [unwired: 3 in, 2 out]
        }
        n25 = Add(x=w119, y=u32 0 ("Address")) -> (x+y=w111:u32)
        n26 = case shown="True" "SMA mode" {
          tunnel: [u8 0 ("In") u8 1 ("In")] -> w124
          frame False {
          }
          frame True {
            # "sma"
          }
        }
        n27 = call "UDP.vi"("In"=w124, "error in (no error)"=w125, "Read (TRUE)"=FALSE, "Address"=w111, "IP address"=w105) -> ("error out"=w112:errorcluster)  [unwired: 3 in, 2 out]
        n28 = Increment(x=w111) -> (x+1=w104:u32)
        n29 = call "UDP.vi"("In"=u8 1, "error in (no error)"=w112, "Read (TRUE)"=FALSE, "Address"=w104, "IP address"=w105) -> ("error out"=w108:errorcluster)  [unwired: 3 in, 2 out]
        n30 = call "UDP.vi"("In"=u8 0, "error in (no error)"=w108, "Read (TRUE)"=FALSE, "Address"=w104, "IP address"=w105) -> ("error out"=w107:errorcluster)  [unwired: 3 in, 2 out]
      }
    }
  }
  n31 = Current VI's Path() -> (path=w95:path)
  n32 = Array Size(array="address") -> (size(s)=w17:i32)
  n33 = Strip Path(path=w95) -> (stripped path=w94:path)  [unwired: 1 out]
  n34 = Multiply(x=w17, y="通道数量") -> (x*y=w14:i32)
  n35 = case shown="True" "use_calib_file" {
    tunnel: w14 -> [w169 _]
    tunnel: [w166 w177] -> w20
    tunnel: [w166 w176] -> w19
    tunnel: [w167 w175] -> w18
    tunnel: w17 -> [_ w174]
    tunnel: "通道数量" -> [_ w173]
    frame False {
      n36 = Initialize Array(u32 0 ("element"), w169) -> (w167:u32[])
      n37 = Initialize Array(u32 0 ("element"), 2048 ("dimension size"), w169) -> (w166:u32[][])
    }
    frame True {
      n38 = call "read_calibration_file_v2.vi"("通道数量"=w173, "板子数量"=w174, "file path (dialog if empty)"="calib_file") -> ("code_density"=w177:i64[][], "accumulation"=w176:u32[][], "Cal Table"=w175:u32[])  [unwired: 5 in, 1 out]
    }
  }
  n39 = case shown="True" FALSE {
    tunnel: w94 -> [w178 w180]
    tunnel: [w178 w179] -> _
    frame False {
    }
    frame True {
      n40 = Build Path(base path=w180, name or relative path="data\\") -> (appended path=w179:path)
    }
  }
  n41 = Format Date/Time String(time format string (%c)="_%Y%m%d_%I%M%S") -> (date/time string=w8:string)  [unwired: 2 in]
  n42 = Concatenate Strings("filename", w8, "_raw.csv") -> (w6:string)
  n43 = local write "pmt trigger rate"(w12) -> ()
  n44 = global write "gloabal.vi" "stop"(w25) -> ()
  n45 = local write "stop"(w25) -> ()
  n46 = for {
    tunnel: "address" -> [w187] mode=indexing
    tunnel: [w186] -> w40 mode=indexing
    tunnel: [w184] -> w39 mode=indexing
    tunnel: w30 -> [w183]
    n47 = TCP Open Connection(address=w187, remote port or service name=u16 24 ("port"), timeout ms (60000)="timeout (ms)", error in (no error)=w183) -> (connection ID=w186:refnum<k5>, error out=w185:errorcluster)  [unwired: 1 in]
    n48 = Merge Errors(w185) -> (w184:errorcluster)
  }
  n49 = Build Path(base path="data  path", name or relative path=w6) -> (appended path=w1:path)
  n50 = Concatenate Strings("filename", w8, ".dat") -> (w93:string)
  n51 = Concatenate Strings("filename", w8, ".csv") -> (w83:string)
  n52 = Concatenate Strings("filename", w8, "_codeDensity" ("string"), ".csv") -> (w76:string)
  n53 = Initialize Array(u32 0 ("element"), w14) -> (w82:u32[])
  n54 = Build Path(base path="data  path", name or relative path=w93) -> (appended path=w92:path)
  "appended path" <- w92
  n55 = Build Path(base path="data  path", name or relative path=w83) -> (appended path=w81:path)
  n56 = Initialize Array(u32 0 ("element"), w14) -> (w13:u32[])
  n57 = call-poly <vilib>:"Write Delimited Spreadsheet.vi"("file path (dialog if empty)"=w1, "2D data"=w4, "append to file? (new file:F)"=FALSE) -> ("new file path (Not A Path if cancelled)"=w2:path)  [unwired: 11 in, 1 out]
  n58 = Multiply(x="factor", y=16) -> (x*y=w56:i32)
  n59 = Initialize Array(u32 0 ("element"), 5000 ("dimension size")) -> (w67:u32[])
  n60 = Build Path(base path="data  path", name or relative path=w76) -> (appended path=w73:path)
  n61 = local write "element"(w11) -> ()
  n62 = for {
    tunnel: [w190] -> w42 mode=indexing
    tunnel: "address" -> [w189] mode=indexing
    (unwired) 2 ("y")
    # "一位数"
    # "两位数"
    n63 = Match Pattern(string=w189, regular expression="." ("search string"), offset (0)=10) -> (after substring=w196:string)  [unwired: 3 out]
    n64 = Decimal String To Number(string=w196) -> (number=w193:i32)  [unwired: 2 in, 1 out]
    n65 = Subtract(x=w193, y=20) -> (x-y=w192:i32)
    n66 = Number To Hexadecimal String(2:w192) -> (0:w195:string)  [unwired: 1 in]
    n67 = String Length(string=w195) -> (length=w201:i32)
    n68 = Divide(x=w201, y=1) -> (x/y=w202:dbl)
    n69 = for {
      N: w202 -> [_]
      shift-right: [w214] -> w191
      shift-left: "" ("format string") -> [w213]
      tunnel: w195 -> [w204]
      i -> [w212]
      w206 = 2 ("y")
      # "字符从ASCII转成16进制表示"
      n70 = Multiply(x=w212, y=w206) -> (x*y=w205:i32)
      n71 = String Subset(string=w204, offset (0)=w205, length (rest)=w206) -> (substring=w207:string)
      n72 = Hexadecimal String To Number(string=w207) -> (number=w211:u32)  [unwired: 2 in, 1 out]
      n73 = Build Array(w211) -> (w210:u32[])
      n74 = To Unsigned Byte Integer(number=w210) -> (unsigned 8bit integer=w209:u8[])
      n75 = Byte Array To String(unsigned byte array=w209) -> (string=w208:string)
      n76 = Concatenate Strings(w213, w208) -> (w214:string)
    }
    n77 = Concatenate Strings("Z", w191) -> (w190:string)
  }
  n78 = Get Date/Time In Seconds() -> (seconds since 1Jan1904=w41:timestamp)
  n79 = Open/Create/Replace File(file path (use dialog)=w92, operation (0:open)=T1."replace or create", access (0:read/write)=enum16{"read/write", "read-only", "write-only"}."write-only", disable buffering (F)=FALSE) -> (refnum out=w97:refnum<file>, error out=w96:errorcluster)  [unwired: 2 in, 1 out]
  n80 = call-poly <vilib>:"Write Delimited Spreadsheet.vi"("file path (dialog if empty)"=w81, "2D data"=w4, "append to file? (new file:F)"=FALSE) -> ("new file path (Not A Path if cancelled)"=w24:path)  [unwired: 11 in, 1 out]
  "csv path" <- w24
  n81 = Initialize Array(0.0, w14) -> (w69:dbl[])
  n82 = Obtain Queue(max queue size (-1, unlimited)=1000000, name (unnamed)="TDC", element data type="TDC" ("name (unnamed)")) -> (queue out=w31:refnum<queue>, error out=→"error out 5":errorcluster)  [unwired: 2 in, 1 out]
  n83 = for {
    tunnel: w40 -> [w221] mode=indexing
    tunnel: w39 -> [w220] mode=indexing
    tunnel: [w219] -> w38 mode=indexing
    tunnel: [w218] -> w37 mode=indexing
    workers-P: _ -> [_]
    tunnel: w31 -> [w217]
    tunnel: [w216] -> w32
    n84 = call "mini.vi"("error in (no error)"=w220, "stop"="stop", "queue out 2"=w217, "connection ID 2"=w221) -> ("error out 3"=w218:errorcluster, "queue out"=w216:refnum<queue>, "connection ID"=w219:refnum<k5>)  [unwired: 5 in]
  }
  n85 = Format Date/Time String(time format string (%c)="%#Y") -> (date/time string=w53:string)  [unwired: 2 in]
  "Year" <- w53
  n86 = Decimal String To Number(string=w53) -> (number=w52:i32)  [unwired: 2 in, 1 out]
  n87 = Number To Hexadecimal String(1:i16 4 ("width (-)"), 2:w52) -> (0:w46:string)
  n88 = String Length(string=w46) -> (length=w48:i32)
  n89 = for {
    tunnel: w38 -> [w224] mode=indexing
    tunnel: w37 -> [w223] mode=indexing
    tunnel: [w222] -> w29
    n90 = TCP Close Connection(connection ID=w224, error in (no error)=w223) -> (error out=w222:errorcluster)  [unwired: 1 in, 1 out]
  }
  n91 = Divide(x=w48, y=2) -> (x/y=w49:dbl)
  n92 = Release Queue(queue=w32) -> (error out=w28:errorcluster)  [unwired: 2 in, 2 out]
  n93 = for {
    N: w49 -> [_]
    shift-right: [w235] -> w45
    shift-left: "" ("format string") -> [w234]
    tunnel: w46 -> [w225]
    i -> [w233]
    w227 = 2 ("y")
    # "字符从ASCII转成16进制表示"
    n94 = Multiply(x=w233, y=w227) -> (x*y=w226:i32)
    n95 = String Subset(string=w225, offset (0)=w226, length (rest)=w227) -> (substring=w228:string)
    n96 = Hexadecimal String To Number(string=w228) -> (number=w232:u32)  [unwired: 2 in, 1 out]
    n97 = Build Array(w232) -> (w231:u32[])
    n98 = To Unsigned Byte Integer(number=w231) -> (unsigned 8bit integer=w230:u8[])
    n99 = Byte Array To String(unsigned byte array=w230) -> (string=w229:string)
    n100 = Concatenate Strings(w234, w229) -> (w235:string)
  }
  n101 = Merge Errors(w29, w28) -> (→"error out 3":errorcluster)
  n102 = case shown="False" "gps" {
    tunnel: w45 -> [_ w237]
    tunnel: ["\u0000" ("format string") w237] -> w44
    frame False {
    }
    frame True {
    }
  }
  n103 = case shown="0, Default" "coarse counter width" {
    tunnel: [u64 549755812864 ("port") u64 288230376151710720 ("port")] -> w22
    frame 0, Default {
    }
    frame 1 {
    }
  }
  n104 = Increment(x="Counter Setting") -> (x+1=w59:dbl)
  n105 = Divide(x=w63, y="Counter Setting") -> (x/y=w62:dbl)
  n106 = while {
    tunnel: w96 -> [w297]
    tunnel: [w278] -> w70
    tunnel: [w267] -> w89
    shift-right: [w294] -> w74
    shift-left: w20 -> [w295]
    tunnel: "Events" -> [w292]
    shift-right: [w291] -> _
    shift-left: w82 -> [w244]
    shift-right: [w290] -> _
    shift-left: u32 0 ("element") -> [w289]
    shift-right: [w288] -> _
    shift-left: w18 -> [w280]
    shift-right: [w282] -> w10
    shift-left: w19 -> [w287]
    tunnel: w24 -> [w274]
    shift-right: [w286] -> _
    shift-left: 0 -> [w261]
    shift-right: [w284] -> _
    shift-left: w41 -> [w283]
    tunnel: w25 -> [_]
    tunnel: w31 -> [w279]
    shift-right: [w275] -> _
    shift-left: w67 -> [w276]
    tunnel: w42 -> [w248]
    tunnel: w63 -> [w272]
    tunnel: w62 -> [w271]
    shift-right: [w266] -> w61
    shift-left: w97 -> [w296]
    tunnel: w59 -> [w265]
    tunnel: w56 -> [w258]
    tunnel: w44 -> [w256]
    tunnel: w41 -> [w255]
    tunnel: "通道数量" -> [w249]
    tunnel: w22 -> [w245]
    shift-right: [w241] -> _
    shift-left: w13 -> [w242]
    tunnel: w12 -> [_]
    tunnel: w11 -> [_]
    tunnel: w2 -> [w240]
    tunnel: w69 -> [w293]
    stop <- w247 stop-if-true
    n107 = local read "save data"() -> (w260:bool)
    n108 = Dequeue Element(queue=w279) -> (element=w251:string, error out=w278:errorcluster)  [unwired: 2 in, 2 out]
    n109 = case shown="True" w260 {
      tunnel: w297 -> [w310 w316]
      tunnel: w296 -> [w311 w315]
      tunnel: w251 -> [_ w314]
      tunnel: [w311 w313] -> w270
      tunnel: [w310 w312] -> w268
      frame False {
      }
      frame True {
        n110 = disable-structure shown="Disabled" {
          disable-tunnel: w316 -> [w323 _]
          disable-tunnel: w315 -> [w322 _]
          disable-tunnel: w314 -> [w319 _]
          disable-tunnel: [w318 _] -> w313
          disable-tunnel: [w317 _] -> w312
          frame Disabled {
            n111 = Write to Binary File(file (use dialog)=w322, data=w319, error in=w323, 5:FALSE ("prepend array or string size? (T)"), 9:T2."big-endian, network order" ("byte order (0:big-endian, network order)")) -> (refnum out=w318:refnum<file>, error out=w317:errorcluster)  [unwired: 1 in, 1 out]
          }
          frame Enabled {
          }
        }
      }
    }
    n112 = String Length(string=w251) -> (length=w262:i32)
    n113 = case shown="True" TRUE {
      tunnel: w283 -> [w335 w345]
      tunnel: [w335 w346] -> w264
      tunnel: w261 -> [w334 w344]
      tunnel: w262 -> [_ w343]
      tunnel: [w334 w342] -> w263
      tunnel: w258 -> [_ w341]
      tunnel: w255 -> [_ w339]
      tunnel: [FALSE w336] -> w254
      frame False {
      }
      frame True {
        n114 = Get Date/Time In Seconds() -> (seconds since 1Jan1904=w340:timestamp)
        n115 = Subtract(x=w340, y=w345) -> (x-y=w348:dbl)
        n116 = Subtract(x=w340, y=w339) -> (x-y=w338:dbl)
        n117 = Greater Or Equal?(x=w338, y="timeout") -> (x >= y?=w336:bool)
        n118 = Greater Or Equal?(x=w348, y=1.0) -> (x >= y?=w349:bool)
        n119 = case shown="True" w349 {
          tunnel: w348 -> [_ w360]
          tunnel: w340 -> [_ w358]
          tunnel: [w353 w358] -> w346
          tunnel: w345 -> [w353 _]
          tunnel: w344 -> [w352 w355]
          tunnel: w343 -> [w351 _]
          tunnel: [w350 0] -> w342
          tunnel: w341 -> [_ w354]
          frame False {
            n120 = Add(x=w351, y=w352) -> (x+y=w350:i32)
          }
          frame True {
            n121 = Divide(x=w355, y=w354) -> (x/y=w357:dbl)
            n122 = Divide(x=w357, y=w360) -> (x/y=→"rate":dbl)
          }
        }
      }
    }
    n123 = local read "display"() -> (w259:bool)
    n124 = case shown="True" w259 {
      tunnel: w251 -> [_ w309]
      frame False {
      }
      frame True {
        "element" <- w309
      }
    }
    n125 = Unbundle By Name(w278) -> ("status"=w277:bool)
    n126 = case shown="True" "display" {
      tunnel: w280 -> [_ w362]
      tunnel: w244 -> [_ w361]
      frame False {
      }
      frame True {
        "Cal Table" <- w362
        "event" <- w361
      }
    }
    n127 = String Length(string=w251) -> (length=w253:i32)
    n128 = local read "stop"() -> (w246:bool)
    n129 = for {
      N: w253 -> [_]
      tunnel: w251 -> [w306]
      tunnel: [w306] -> w252
      tunnel: [w305] -> w250
      tunnel: w248 -> [w303]
      i -> [w305]
      stop <- w299 stop-if-true
      n130 = Index Array(array=w303) -> (element=w304:string)  [unwired: 1 in]
      n131 = Index Array(array=w303, index=1) -> (element=w301:string)
      n132 = String Subset(string=w306, offset (0)=w305, length (rest)=2 ("length (rest)")) -> (substring=w300:string)
      n133 = Equal?(x=w300, y=w304) -> (x = y?=w307:bool)
      n134 = Equal?(x=w300, y=w301) -> (x = y?=w298:bool)
      n135 = Or(x=w307, y=w298) -> (x .or. y?=w299:bool)
    }
    n136 = case shown="True" "replace dat" {
      tunnel: w270 -> [w325 w331]
      tunnel: [w325 w330] -> w266
      tunnel: w268 -> [w324 w327]
      tunnel: [w324 w326] -> w267
      frame False {
      }
      frame True {
        n137 = Close File(refnum=w331, error in=w327) -> (path=w332:path, error out=w328:errorcluster)
        n138 = Open/Create/Replace File(file path (use dialog)=w332, error in=w328, operation (0:open)=T1."replace or create") -> (refnum out=w330:refnum<file>, error out=w326:errorcluster)  [unwired: 3 in, 1 out]
      }
    }
    n139 = Greater Or Equal?(x=w289, y=w292) -> ()  [unwired: 1 out]
    n140 = Compound Arithmetic op=OR(FALSE ("x"), w277, w254, w246) -> (w247:bool)
    n141 = String Subset(string=w252, offset (0)=w250) -> (substring=w243:string)  [unwired: 1 in]
    n142 = global write "gloabal.vi" "stop"(w247) -> ()
    n143 = while {
      tunnel: w243 -> [w384]
      shift-right: [w453] -> w294
      shift-left: w295 -> [w451]
      shift-right: [w447] -> w291
      shift-left: w244 -> [w446]
      tunnel: [w445] -> w290
      tunnel: w289 -> [w444]
      shift-right: [w442] -> w288
      shift-left: w280 -> [w443]
      tunnel: w274 -> [w440]
      shift-right: [w439] -> w282
      shift-left: w287 -> [w409]
      shift-right: [w436] -> w275
      shift-left: w276 -> [w437]
      tunnel: w243 -> [w403]
      tunnel: w272 -> [w416]
      tunnel: w271 -> [w415]
      tunnel: w265 -> [w408]
      tunnel: w256 -> [w398]
      tunnel: w249 -> [w386]
      tunnel: w248 -> [w385]
      tunnel: w245 -> [w381]
      tunnel: w243 -> [w371]
      shift-right: [w373] -> w241
      shift-left: w242 -> [w375]
      tunnel: w240 -> [w367]
      tunnel: w293 -> [w450]
      i -> [w454]
      stop <- w411 stop-if-true
      (unwired) 10 ("length (rest)")
      (unwired) u64 8323072 ("port")
      (unwired) i16 -16 ("y")
      n144 = Multiply(x=w454, y=16 ("length (rest)")) -> (x*y=w376:i32)
      n145 = local read "display"() -> (w438:bool)
      n146 = Add(x=w376, y=8 ("length (rest)")) -> (x+y=w428:i32)
      n147 = Add(x=w376, y=7 ("length (rest)")) -> (x+y=w405:i32)
      n148 = Add(x=w376, y=3 ("length (rest)")) -> (x+y=w378:i32)
      n149 = Add(x=w376, y=0 ("length (rest)")) -> (x+y=w414:i32)
      n150 = String Subset(string=w384, offset (0)=0, length (rest)=2 ("length (rest)")) -> (substring=w387:string)
      "name (unnamed)" <- w387
      n151 = String Subset(string=w384, offset (0)=w414, length (rest)=16 ("y")) -> (substring=w412:string)
      n152 = String Subset(string=w384, offset (0)=w414, length (rest)=8 ("length (rest)")) -> (substring=w396:string)
      n153 = String Subset(string=w403, offset (0)=w428, length (rest)=8 ("length (rest)")) -> (substring=w393:string)
      n154 = String Subset(string=w403, offset (0)=w405, length (rest)=4 ("length (rest)")) -> (substring=w392:string)
      n155 = Search 1D Array(1D array=w385, element=w387) -> (index of element=w388:i32)  [unwired: 1 in]
      n156 = case shown="True" w438 {
        tunnel: w451 -> [_ w500]
        frame False {
        }
        frame True {
          n157 = Index Array(array=w500, index (col)="channel for cal") -> (element=→"cal":i64[])  [unwired: 1 in]
        }
      }
      n158 = String Subset(string=w371, offset (0)=w378, length (rest)=4 ("length (rest)")) -> (substring=w369:string)
      n159 = String Length(string=w412) -> (length=w449:i32)
      n160 = Less?(x=w449, y=16) -> (x < y?=w411:bool)
      n161 = String Subset(string=w396, length (rest)=1 ("length (rest)")) -> (substring=w433:string)  [unwired: 1 in]
      n162 = String Subset(string=w396, offset (0)=7, length (rest)=1 ("length (rest)")) -> (substring=w417:string)
      n163 = Multiply(x=w388, y=w386) -> (x*y=w382:i32)
      n164 = Not Equal?(x="", y=w369) -> (x != y?=w370:bool)
      n165 = String Subset(string=w396, offset (0)=2, length (rest)=1 ("length (rest)")) -> (substring=w394:string)
      n166 = Equal?(x=w433, y="Z" ("format string")) -> (x = y?=w419:bool)
      n167 = Equal?(x=w417, y=w398) -> (x = y?=w418:bool)
      n168 = String To Byte Array(string=w393) -> (unsigned byte array=w425:u8[])
      n169 = String To Byte Array(string=w392) -> (unsigned byte array=w399:u8[])
      n170 = String To Byte Array(string=w394) -> (unsigned byte array=w456:u8[])
      n171 = for {
        shift-right: [w671] -> w422
        shift-left: "" ("format string") -> [w668]
        tunnel: w456 -> [w672] mode=indexing
        n172 = Number To Hexadecimal String(2:w672) -> (0:w664:string)  [unwired: 1 in]
        n173 = String Length(string=w664) -> (length=w670:i32)
        n174 = Equal?(x=w670, y=2) -> (x = y?=w667:bool)
        n175 = Concatenate Strings("0" ("format string"), w664) -> (w666:string)
        n176 = Select(t=w664, s=w667, f=w666) -> (s? t:f=w663:string)
        n177 = Concatenate Strings(w668, w663) -> (w671:string)
      }
      n178 = for {
        shift-right: [w496] -> w423
        shift-left: "" ("format string") -> [w488]
        tunnel: w425 -> [w497] mode=indexing
        n179 = Number To Hexadecimal String(2:w497) -> (0:w490:string)  [unwired: 1 in]
        n180 = String Length(string=w490) -> (length=w495:i32)
        n181 = Concatenate Strings("0" ("format string"), w490) -> (w492:string)
        n182 = Equal?(x=w495, y=2) -> (x = y?=w493:bool)
        n183 = Select(t=w490, s=w493, f=w492) -> (s? t:f=w489:string)
        n184 = Concatenate Strings(w488, w489) -> (w496:string)
      }
      n185 = for {
        shift-right: [w486] -> w402
        shift-left: "" ("format string") -> [w478]
        tunnel: w399 -> [w487] mode=indexing
        n186 = Number To Hexadecimal String(2:w487) -> (0:w480:string)  [unwired: 1 in]
        n187 = String Length(string=w480) -> (length=w485:i32)
        n188 = Concatenate Strings("0" ("format string"), w480) -> (w482:string)
        n189 = Equal?(x=w485, y=2) -> (x = y?=w483:bool)
        n190 = Select(t=w480, s=w483, f=w482) -> (s? t:f=w479:string)
        n191 = Concatenate Strings(w478, w479) -> (w486:string)
      }
      n192 = Not(x=w411) -> (.not. x?=w410:bool)
      n193 = Compound Arithmetic op=AND(w419, w418, w410) -> (w431:bool)
      n194 = Hexadecimal String To Number(string=w422, default (0uL)=u64 0 ("default (0 U32)")) -> (number=w452:u64)  [unwired: 1 in, 1 out]
      n195 = Hexadecimal String To Number(string=w423, default (0uL)=u64 0 ("default (0 U32)")) -> (number=w391:u64)  [unwired: 1 in, 1 out]
      n196 = Hexadecimal String To Number(string=w402, default (0uL)=u64 0 ("default (0 U32)")) -> (number=w380:u64)  [unwired: 1 in, 1 out]
      n197 = And(x=w452, y=u64 127 ("port")) -> (x .and. y?=w383:u64)
      "channel number" <- w383
      n198 = Add(x=w382, y=w383) -> (x+y=w374:u64)
      n199 = case shown="True" w370 {
        tunnel: w375 -> [w458 w464]
        tunnel: w374 -> [_ w462]
        tunnel: [w458 w461] -> w373
        tunnel: w369 -> [_ w460]
        frame False {
        }
        frame True {
          n200 = String To Byte Array(string=w460) -> (unsigned byte array=w465:u8[])
          n201 = for {
            shift-right: [w476] -> w459
            shift-left: "" ("format string") -> [w468]
            tunnel: w465 -> [w477] mode=indexing
            n202 = Number To Hexadecimal String(2:w477) -> (0:w470:string)  [unwired: 1 in]
            n203 = String Length(string=w470) -> (length=w475:i32)
            n204 = Concatenate Strings("0" ("format string"), w470) -> (w472:string)
            n205 = Equal?(x=w475, y=2) -> (x = y?=w473:bool)
            n206 = Select(t=w470, s=w473, f=w472) -> (s? t:f=w469:string)
            n207 = Concatenate Strings(w468, w469) -> (w476:string)
          }
          n208 = Hexadecimal String To Number(string=w459, default (0uL)=u64 0 ("default (0 U32)")) -> (number=w463:u64)  [unwired: 1 in, 1 out]
          n209 = Replace Array Subset(array=w464, new element=w463, index=w462) -> (w461:u32[])
        }
      }
      n210 = case shown="True" w431 {
        tunnel: w391 -> [_ w509]
        tunnel: w444 -> [w504 w524]
        tunnel: w451 -> [w506 w532]
        tunnel: [w506 w531] -> w453
        tunnel: w450 -> [_ w528]
        tunnel: w374 -> [_ w514]
        tunnel: w446 -> [w505 w527]
        tunnel: [w505 w526] -> w447
        tunnel: [w504 w525] -> w445
        tunnel: w443 -> [w503 w523]
        tunnel: [w503 w522] -> w442
        tunnel: w409 -> [w502 w520]
        tunnel: [w502 w519] -> w439
        tunnel: w440 -> [_ w518]
        tunnel: w437 -> [w501 w516]
        tunnel: [w501 w515] -> w436
        tunnel: w416 -> [_ w513]
        tunnel: w415 -> [_ w512]
        tunnel: w408 -> [_ w511]
        tunnel: w380 -> [_ w510]
        tunnel: w381 -> [_ w508]
        tunnel: w367 -> [_ w507]
        frame False {
          (unwired) FALSE
        }
        frame True {
          n211 = Index Array(array=w523, index=w514) -> (element=w521:u32)
          n212 = Greater?(x=w521, y=w511) -> (0:w517:bool)
          n213 = And(x=w509, y=u64 1023 ("port")) -> (x .and. y?=w529:u64)
          n214 = case shown="True" w517 {
            tunnel: w532 -> [w547 w629]
            tunnel: [w546 w629] -> w531
            tunnel: w529 -> [w539 w591]
            tunnel: w528 -> [_ w579]
            tunnel: w524 -> [w544 _]
            tunnel: w514 -> [w542 w581]
            tunnel: w527 -> [w545 w635]
            tunnel: [w545 w634] -> w526
            tunnel: [w544 w632] -> w525
            tunnel: w521 -> [w540 _]
            tunnel: w523 -> [w543 w631]
            tunnel: [w541 w631] -> w522
            tunnel: w521 -> [w537 _]
            tunnel: w511 -> [w534 _]
            tunnel: w520 -> [w536 w621]
            tunnel: [w535 w621] -> w519
            tunnel: w518 -> [_ w620]
            tunnel: w516 -> [w533 w617]
            tunnel: [w533 w616] -> w515
            tunnel: w514 -> [_ w613]
            tunnel: w513 -> [_ w611]
            tunnel: w512 -> [_ w612]
            tunnel: w510 -> [_ w606]
            tunnel: w510 -> [_ w595]
            tunnel: w509 -> [_ w578]
            tunnel: w508 -> [_ w589]
            tunnel: w507 -> [_ w582]
            frame False {
              n215 = Equal?(x=w537, y=w534) -> (x = y?=w538:bool)
              n216 = case shown="False" w538 {
                tunnel: w547 -> [w558 w564]
                tunnel: [w556 w564] -> w546
                tunnel: w543 -> [w554 w562]
                tunnel: w542 -> [w553 w559]
                tunnel: [w551 w561] -> w541
                tunnel: w540 -> [w550 w560]
                tunnel: w539 -> [w549 _]
                tunnel: w536 -> [w548 w566]
                tunnel: [w548 w565] -> w535
                frame False {
                  n217 = Index Array(array=w558, index (row)=w549, index (col)=w553) -> (element=w557:i64)
                  n218 = Increment(x=w557) -> (x+1=w555:i64)
                  n219 = Replace Array Subset(array=w558, new element=w555, index (row)=w549, index (col)=w553) -> (w556:i64[][])
                  n220 = Increment(x=w550) -> (x+1=w552:u32)
                  n221 = Replace Array Subset(array=w554, new element=w552, index=w553) -> (w551:u32[])
                  "Calibration Counter" <- w550
                }
                frame True {
                  n222 = for {
                    N: 2048 -> [_]
                    tunnel: w564 -> [w576]
                    tunnel: w559 -> [w569]
                    shift-right: [w571] -> w565
                    shift-left: w566 -> [w572]
                    i -> [w568]
                    n223 = Array Subset(array=w576, index (row)=0 ("索引"), length (row)=w568, index (col)=w569, length (col)=1 ("长度")) -> (w573:i64[][])
                    n224 = Add Array Elements(numeric array=w573) -> (sum=w570:i64)
                    n225 = Replace Array Subset(array=w572, new element=w570, index (row)=w568, index (col)=w569) -> (w571:u32[][])
                  }
                  n226 = Increment(x=w560) -> (x+1=w563:u32)
                  n227 = Replace Array Subset(array=w562, new element=w563, index=w559) -> (w561:u32[])
                }
              }
            }
            frame True {
              (unwired) 0.0 ("x")
              w626 = 0 ("索引 (行)")
              w628 = 1 ("长度")
              # "正式取数"
              n228 = And(x=w595, y=u64 126976 ("port")) -> (x .and. y?=w603:u64)
              n229 = And(x=w606, y=u64 4032 ("port")) -> (x .and. y?=w609:u64)
              n230 = Logical Shift(y=i16 -6, x=w609) -> (x << y=w592:u64)
              n231 = Logical Shift(y=i16 -12, x=w603) -> (x << y=w602:u64)
              n232 = And(x=w595, y=u64 63 ("port")) -> (x .and. y?=w585:u64)
              n233 = And(x=w578, y=w589) -> (x .and. y?=w590:u64)
              n234 = Multiply(x=u64 3600, y=w602) -> (x*y=w598:u64)
              n235 = Multiply(x=u64 60, y=w592) -> (x*y=w599:u64)
              n236 = Logical Shift(y=i16 -10, x=w590) -> (x << y=w587:u64)
              "coarse" <- w587
              n237 = Add(x=w599, y=w598) -> (x+y=w597:u64)
              n238 = Add(x=w597, y=w585) -> (x+y=w588:u64)
              "second stamp" <- w588
              n239 = Add(x=w587, y=w588) -> (x+y=w586:u64)
              n240 = Equal?(x=w613, y=u32 2) -> (x = y?=w615:bool)
              n241 = case shown="True" w615 {
                tunnel: w617 -> [w640 w643]
                tunnel: w586 -> [_ w642]
                tunnel: [w640 w641] -> w616
                frame False {
                }
                frame True {
                  n242 = Build Array (concatenate)(w643, w642) -> (w641:u64[])
                }
              }
              "cal 2" <- w616
              n243 = case shown="True" TRUE {
                tunnel: [w650 w658] -> w637
                tunnel: w629 -> [_ _]
                tunnel: w581 -> [w655 w656]
                tunnel: w591 -> [w653 w661]
                tunnel: w621 -> [w654 w662]
                frame False {
                  w649 = 0 ("index (row)")
                  w652 = 1 ("长度")
                  n244 = Decrement(x=w655) -> (x-1=w648:u64)
                  n245 = Array Subset(array=w654, index (row)=w653, length (row)=w652, index (col)=w648, length (col)=w652) -> (w651:u32[][])
                  n246 = Index Array(array=w651, index (row)=w649, index (col)=w649) -> (element=w650:u32)
                }
                frame True {
                  w657 = 0 ("index (row)")
                  w660 = 1 ("长度")
                  n247 = Array Subset(array=w662, index (row)=w661, length (row)=w660, index (col)=w656, length (col)=w660) -> (w659:u32[][])
                  n248 = Index Array(array=w659, index (row)=w657, index (col)=w657) -> (element=w658:u32)
                }
              }
              n249 = Multiply(x=w586, y=w611) -> (x*y=w577:dbl)
              n250 = Index Array(array=w635, index=w581) -> (element=w632:u32)
              n251 = Array Subset(array=w629, index (row)=w591, length (row)=w628, index (col)=w581, length (col)=w628) -> (w627:i64[][])
              n252 = Index Array(array=w627, index (row)=w626, index (col)=w626) -> (element=w625:i64)
              n253 = Divide(x=w625, y=u32 2) -> (x/y=w630:dbl)
              n254 = Increment(x=w632) -> (x+1=w633:u32)
              n255 = Add(x=w637, y=w630) -> (x+y=w636:dbl)
              n256 = Add(x=w577, y=0.0) -> (x+y=w594:dbl)
              n257 = Multiply(x=w636, y=w612) -> (x*y=w623:dbl)
              n258 = Replace Array Subset(array=w579, new element=w578, index=w581) -> (w580:dbl[])
              n259 = Subtract(x=w611, y=w623) -> (x-y=w610:dbl)
              n260 = Add(x=w610, y=w594) -> (x+y=w624:dbl)
              n261 = Replace Array Subset(array=w635, new element=w633, index=w581) -> (w634:u32[])
              n262 = Replace Array Subset(array=w579, new element=w624, index=w581) -> (w619:dbl[])
              n263 = case shown="True" "save data" {
                tunnel: w620 -> [_ w647]
                tunnel: w619 -> [_ w645]
                frame False {
                }
                frame True {
                  n264 = call-poly <vilib>:"Write Delimited Spreadsheet.vi"("file path (dialog if empty)"=w647, "1D data"=w645, "append to file? (new file:F)"="append csv", "delimiter (\\t)"="," ("delimiter (\\t)")) -> ()  [unwired: 10 in, 2 out]
                }
              }
              n265 = call-poly <vilib>:"Write Delimited Spreadsheet.vi"("file path (dialog if empty)"=w582, "1D data"=w580, "append to file? (new file:F)"="append csv 2", "delimiter (\\t)"="," ("delimiter (\\t)")) -> ()  [unwired: 10 in, 2 out]
              "fine" <- w591
            }
          }
        }
      }
      n266 = Decimate 1D Array(w373) -> (→"pmt trigger rate":u32[])  [unwired: 1 out]
    }
    n267 = case shown="False" "RST" {
      tunnel: w263 -> [w364 _]
      tunnel: [w364 0] -> w286
      tunnel: [w363 w365] -> w284
      tunnel: w264 -> [w363 _]
      frame False {
      }
      frame True {
        n268 = Get Date/Time In Seconds() -> (seconds since 1Jan1904=w365:timestamp)
      }
    }
  }
  "error out 2" <- w70
  "accumulation" <- w10
  n269 = Close File(refnum=w61, error in=w89) -> (error out=→"error out":errorcluster)  [unwired: 1 out]
  n270 = call-poly <vilib>:"Write Delimited Spreadsheet.vi"("file path (dialog if empty)"=w73, "2D data"=w74, "append to file? (new file:F)"=FALSE, "transpose? (no:F)"=TRUE, "delimiter (\\t)"="," ("delimiter (\\t)")) -> ()  [unwired: 9 in, 2 out]
